vi "界面UI.vi"() -> ()   [LabVIEW 2016, in "超标留样集成.lvlib" / "ESTD1200.lvlib"]
uses:
  ESTD1200.lvlib
  <vilib>/Utility/miscctls.llb/LVPointTypeDef.ctl
  <vilib>/Plasmionique/MB Master/MB_Master/MB_Master.lvclass
  <vilib>/ptbypt/NI_PtbyPt.lvlib
  <vilib>/Plasmionique/MB Master/MB Master.lvlib
panel:
  in  "清除告警":bool
  in  "开门":bool
  out "采样瓶状态":T1
  out "冰箱温度":sgl
  out "瓶数":u16
  out "当前进程":u16(ring) items=["待机", "电机复位", "采样瓶转到采样区", "采样瓶排空", "采样泵管润洗", "采样瓶再排空", "采样", "采样泵反转排空管路", "取样瓶转到取样区"]
  out "流程计时/s":i32
  in  "设置":bool
  out "单次采样量":u16
  out "留样模式":enum16{"定时采样", "外控采样", "时间等比", "流量等比", "液位等比"}(ring)
  out "门状态":enum16{"门开", "门关"}(ring)
  out "报警状态":T2(ring)
  out "仪器时间":timestamp format="%<%Y/%m/%d %H:%M:%S>T"
  out "当前瓶号":u16
  out "采样器状态":enum16{"空闲", "忙碌"}(ring)
  out "采样器进程":i32(listbox)
  out "流程中":bool
  in  "停止流程":bool
  in  "启动流程":bool
  in  "远程复位":bool
  in  "远程留样":bool
  in  "停止命令":bool
  out "通讯":bool
  # "德润DR803L超标留样"
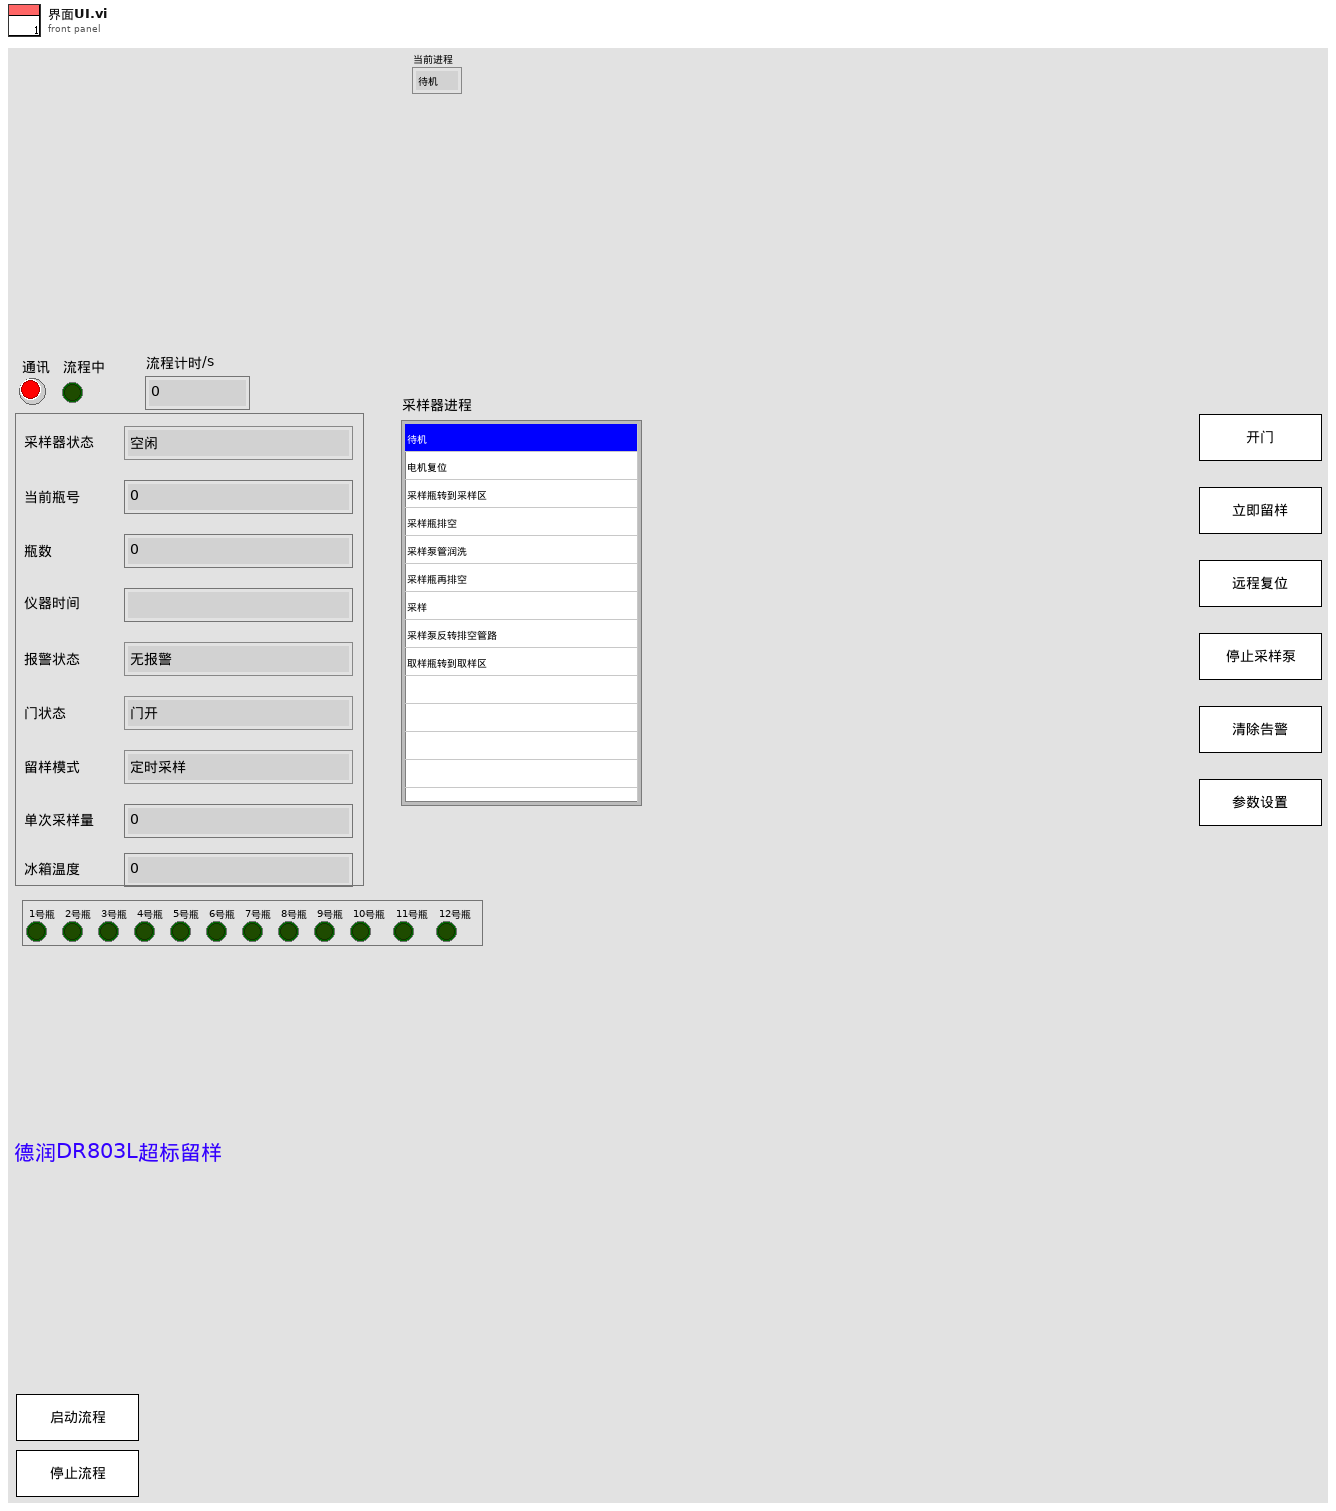
[diagram p1: front panel]
types:
  T1 = typedef "留样瓶状态.ctl" = cluster{"1号瓶":bool, "2号瓶":bool, "3号瓶":bool, "4号瓶":bool, "5号瓶":bool, "6号瓶":bool, "7号瓶":bool, "8号瓶":bool, "9号瓶":bool, "10号瓶":bool, "11号瓶":bool, "12号瓶":bool}
  T2 = enum16{"无报警", "通讯异常(采样器与工控机通讯)", "滑台电机异常(过温/过流)", "蠕动泵异常(过温/过流)", "转盘电机异常(过温/过流)", "编码器异常", "转盘原点传感器异常", "滑台原点传感器异常", "冰箱温度异常", "冰箱通讯异常", "门禁锁异常", "串口屏通信异常", "SD卡异常告警", "Flash异常告警(W25Q32)", "留样失败", "瓶满告警", "复位异常"}
  T3 = typedef "队列data.ctl" = cluster{"命令":string, "data":cluster{"站号":u16, "控制命令":u16[]}}
  T4 = cluster{"STEP":enum16{"open", "read", "write", "write single", "close"}, "starting address":u16, "value":u16}
  T5 = typedef "LVPointTypeDef.ctl" = cluster{"Horizontal":i16, "Vertical":i16}
  T6 = cluster{"命令":string, "data":cluster{"站号":u16, "控制命令":u16[]}}
  T7 = enum16{"open", "read", "write", "write single", "close"}
  T8 = enum32{"Bad", "Idle", "Run top level", "Running"}
  T9 = cluster{"当前瓶号":u16, "瓶数":u16, "采样量":u16, "采样模式":u16, "整点定时时间":cluster{"1":bool, "2":bool, "3":bool, "4":bool, "5":bool, "6":bool, "7":bool, "8":bool, "9":bool, "10":bool, "11":bool, "12":bool, "13":bool, "14":bool, "15":bool, "16":bool, "17":bool, "19":bool, "19":bool, "20":bool, "21":bool, "22":bool, "23":bool, "24":bool}, "氨氮":sgl, "总磷":sgl, "总氮":sgl, "CODMn":sgl, "CODCr":sgl, "PH":sgl, "溶解氧":sgl, "时间等比采样间隔":u16, "流量等比采样间隔":sgl, "4mA流量":sgl, "20mA流量":sgl, "当前流量":sgl, "液位等比采样间隔":sgl, "4mA液位":sgl, "20mA液位":sgl, "当前液位":sgl}
  T10 = cluster{"1":bool, "2":bool, "3":bool, "4":bool, "5":bool, "6":bool, "7":bool, "8":bool, "9":bool, "10":bool, "11":bool, "12":bool, "13":bool, "14":bool, "15":bool, "16":bool, "17":bool, "19":bool, "19":bool, "20":bool, "21":bool, "22":bool, "23":bool, "24":bool}
  T11 = cluster{"采样器状态":u16, "采样模式":u16, "瓶数":u16, "采样量":u16, "当前瓶号":u16, "当前进程":u16, "采样瓶状态":cluster{"1号瓶":bool, "2号瓶":bool, "3号瓶":bool, "4号瓶":bool, "5号瓶":bool, "6号瓶":bool, "7号瓶":bool, "8号瓶":bool, "9号瓶":bool, "10号瓶":bool, "11号瓶":bool, "12号瓶":bool}, "门锁状态":bool, "冰箱当前温度":sgl, "系统时间":timestamp}
  T12 = cluster{"系统时间":timestamp, "当前进程":u16, "采样模式":u16, "告警代码":u16, "故障代码":u16, "软件版本":string}
  T13 = cluster{"1号瓶":bool, "2号瓶":bool, "3号瓶":bool, "4号瓶":bool, "5号瓶":bool, "6号瓶":bool, "7号瓶":bool, "8号瓶":bool, "9号瓶":bool, "10号瓶":bool, "11号瓶":bool, "12号瓶":bool}
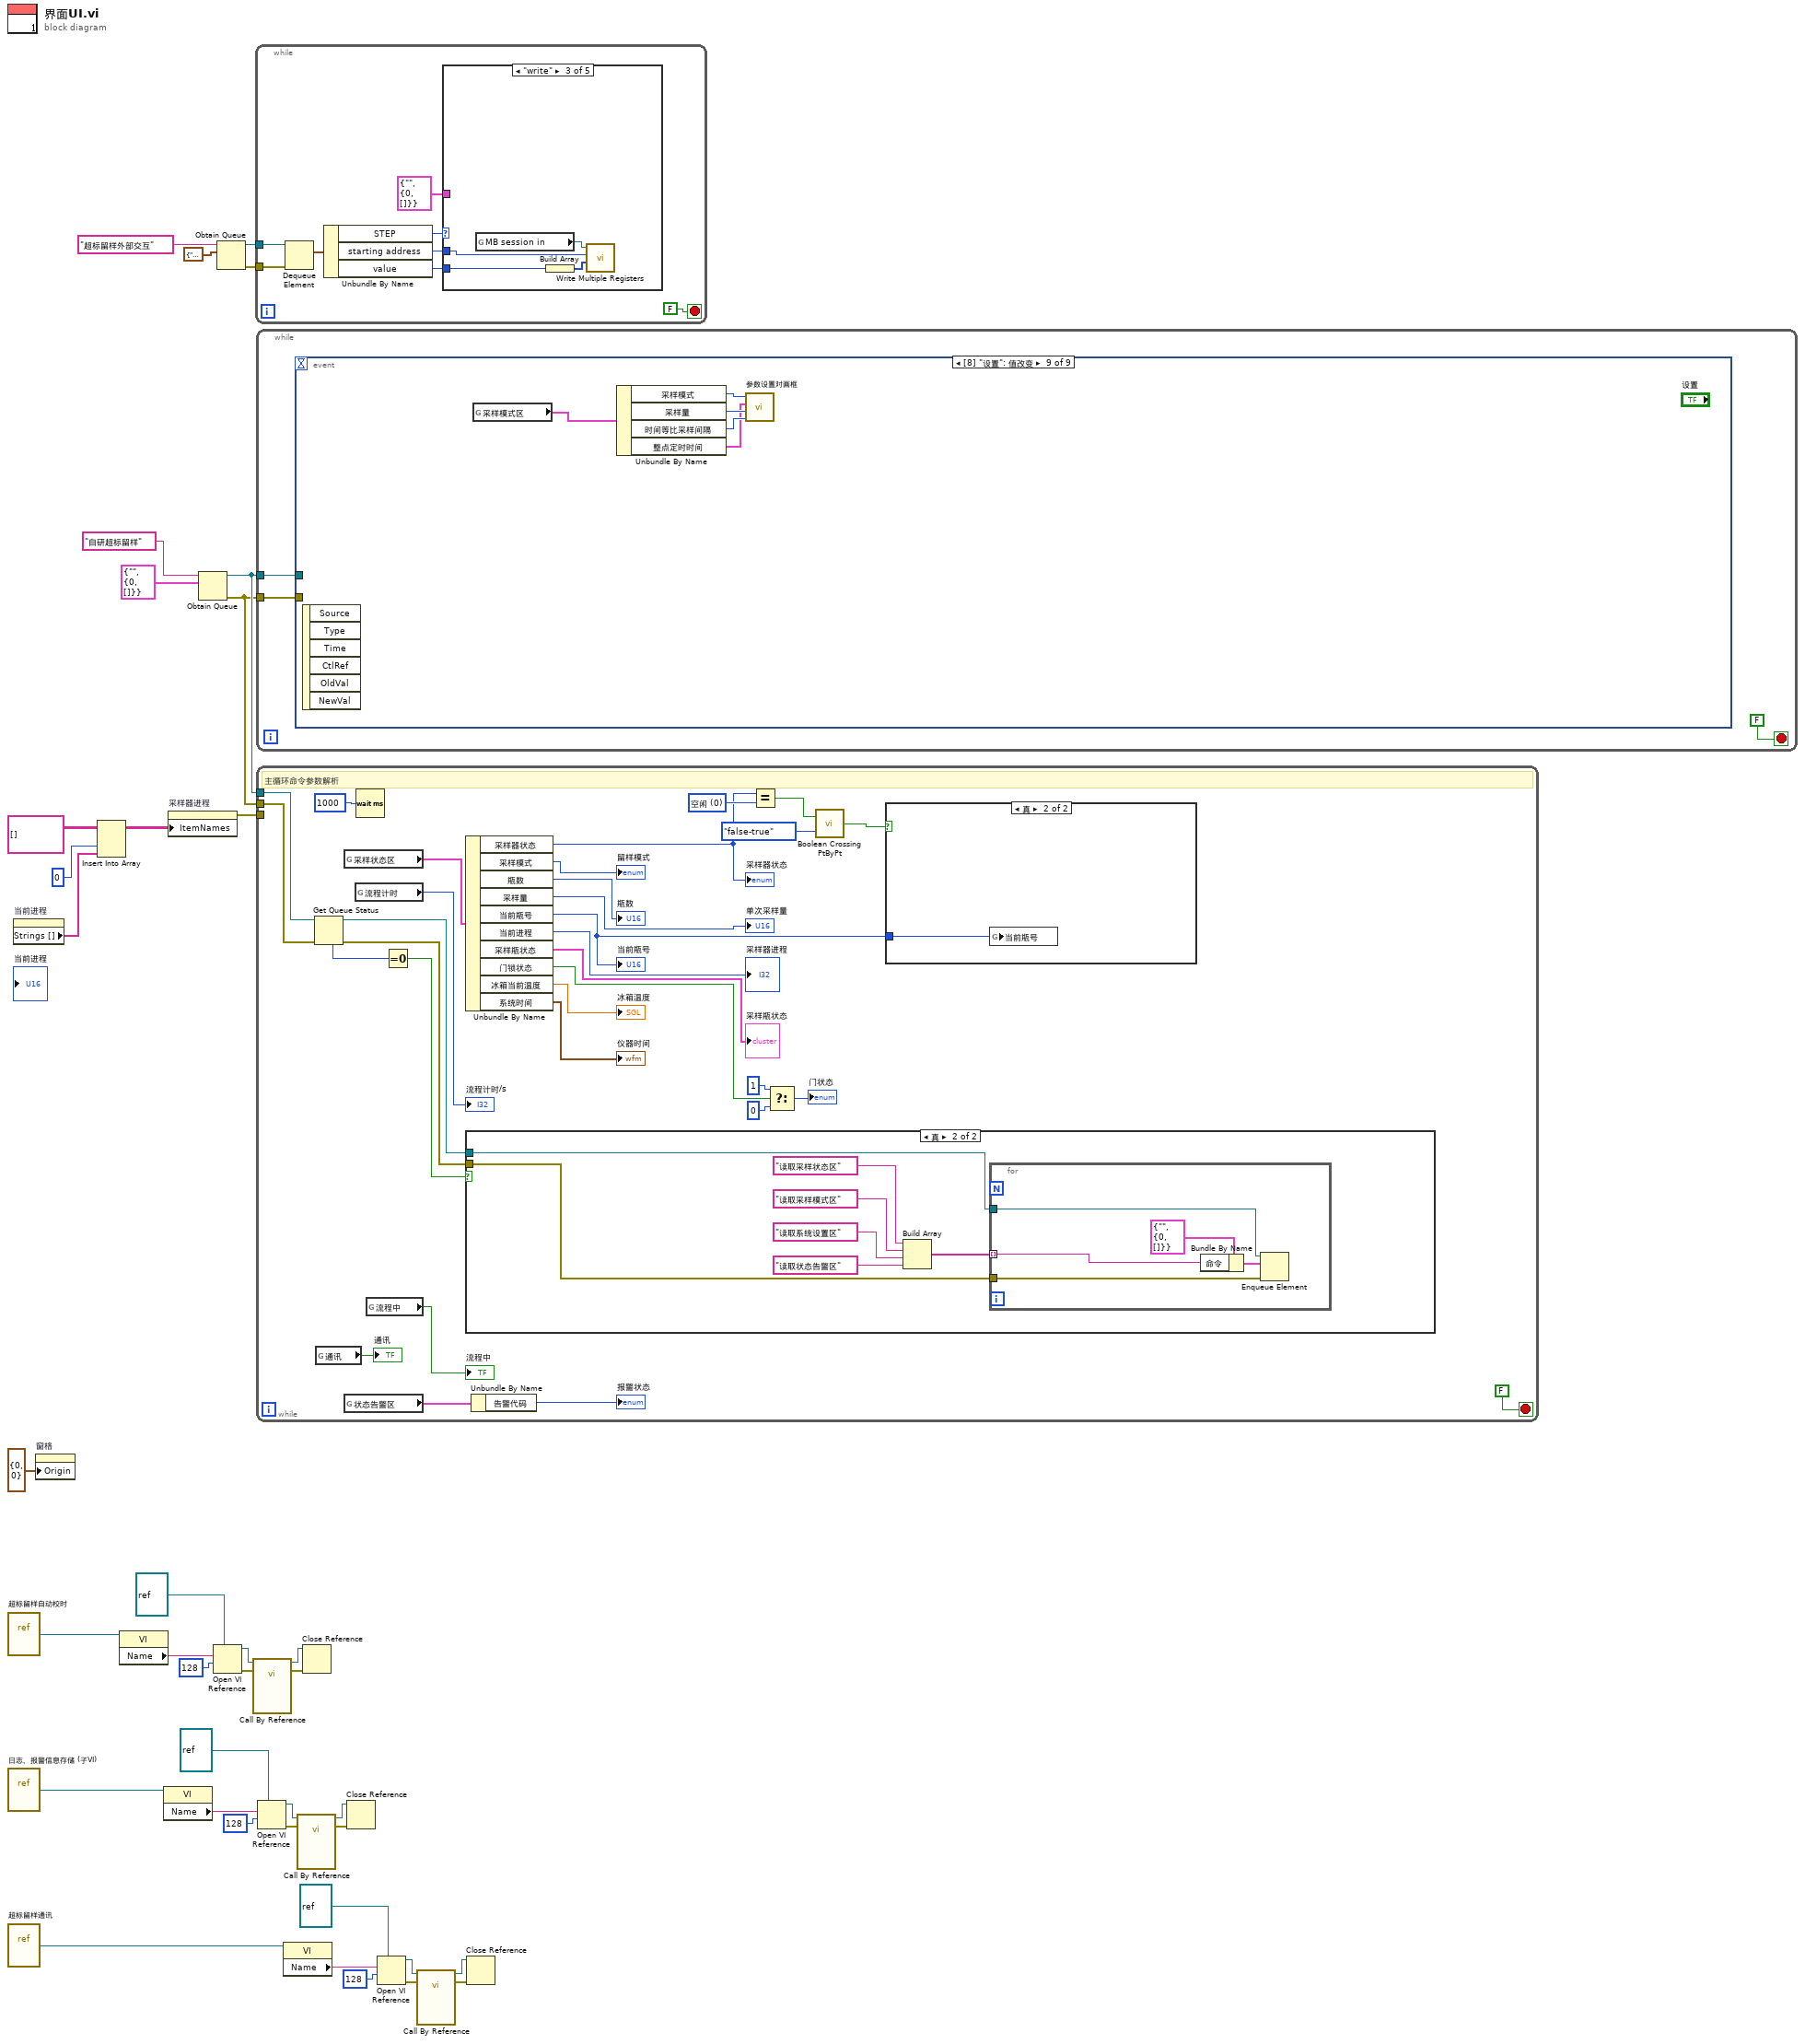
[diagram p0: block diagram]
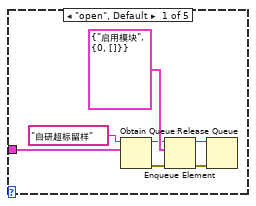
[diagram p2: hidden frame]
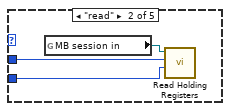
[diagram p3: hidden frame]
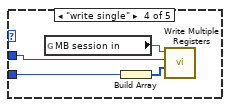
[diagram p4: hidden frame]
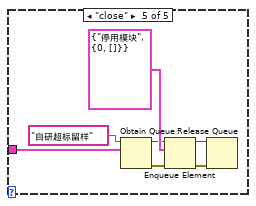
[diagram p5: hidden frame]
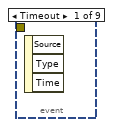
[diagram p6: hidden frame]
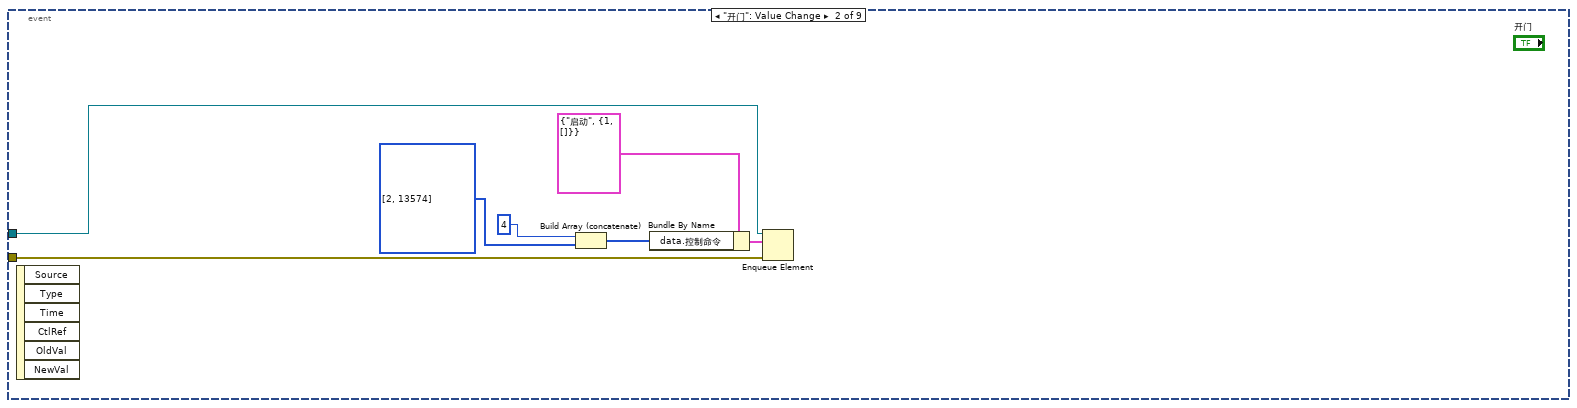
[diagram p7: hidden frame]
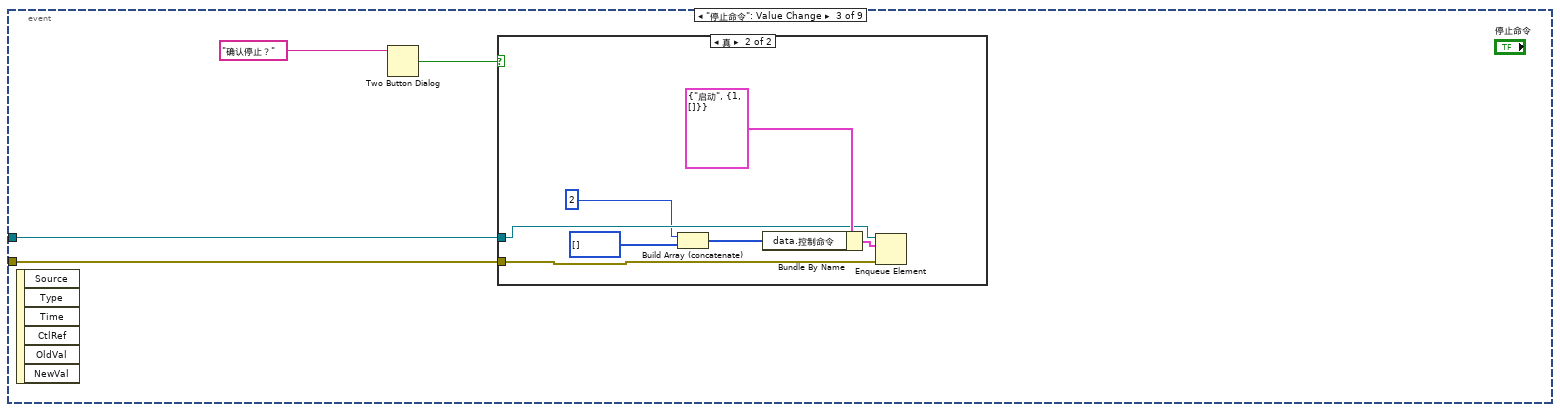
[diagram p8: hidden frame]
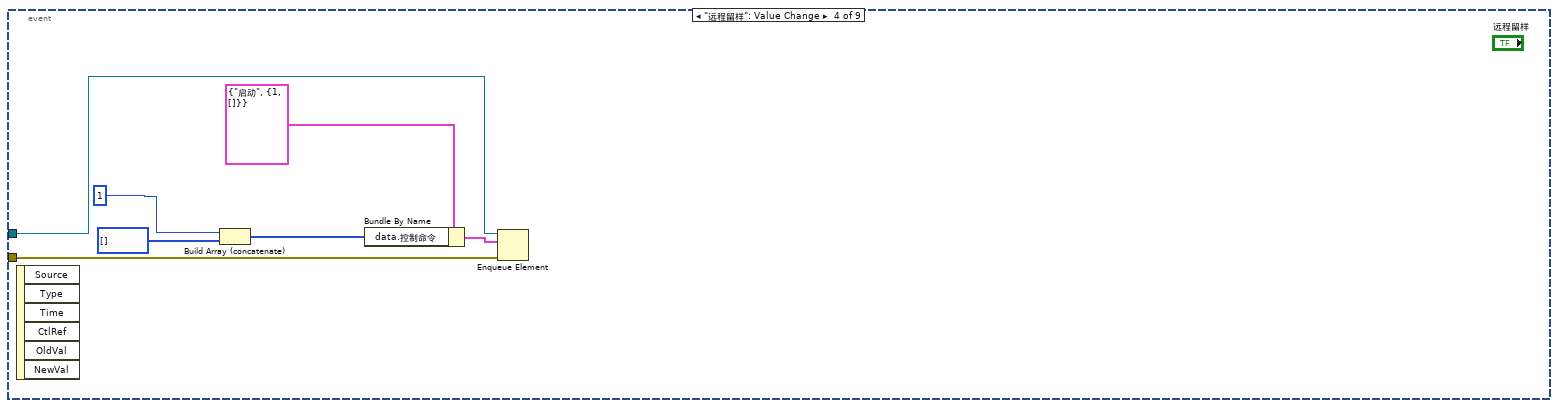
[diagram p10: hidden frame]
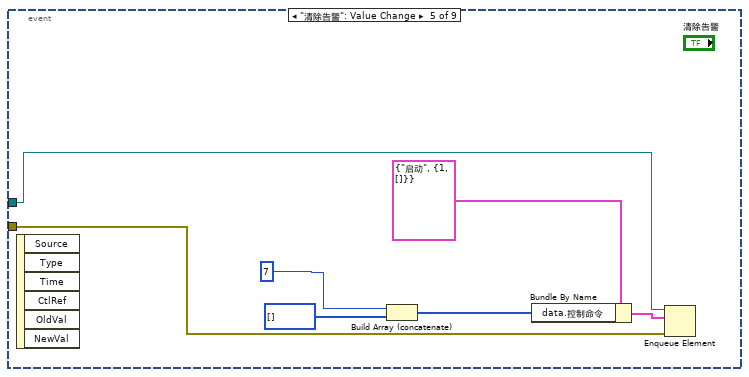
[diagram p11: hidden frame]
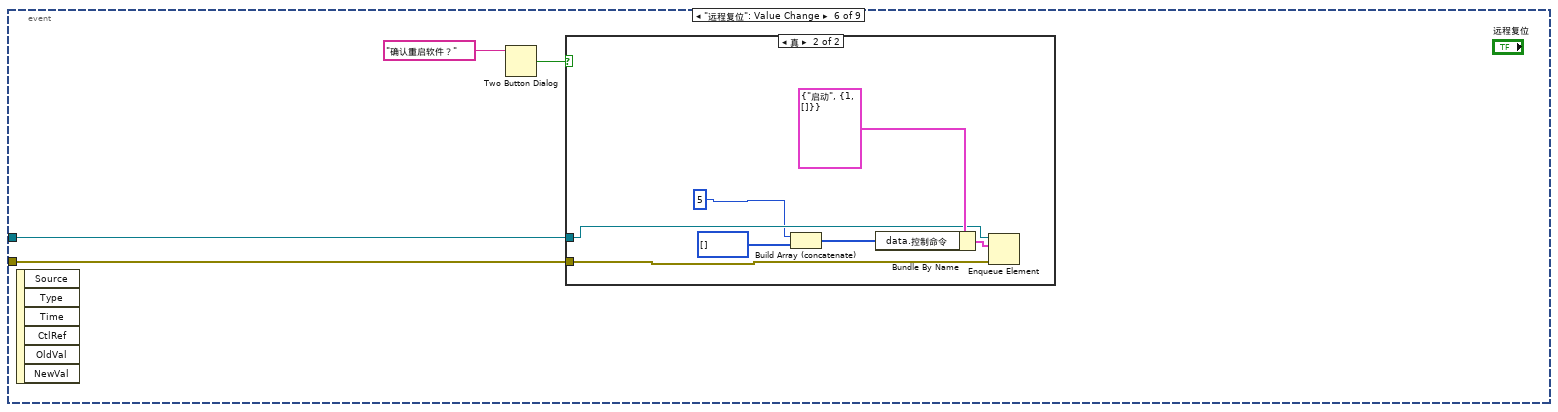
[diagram p12: hidden frame]
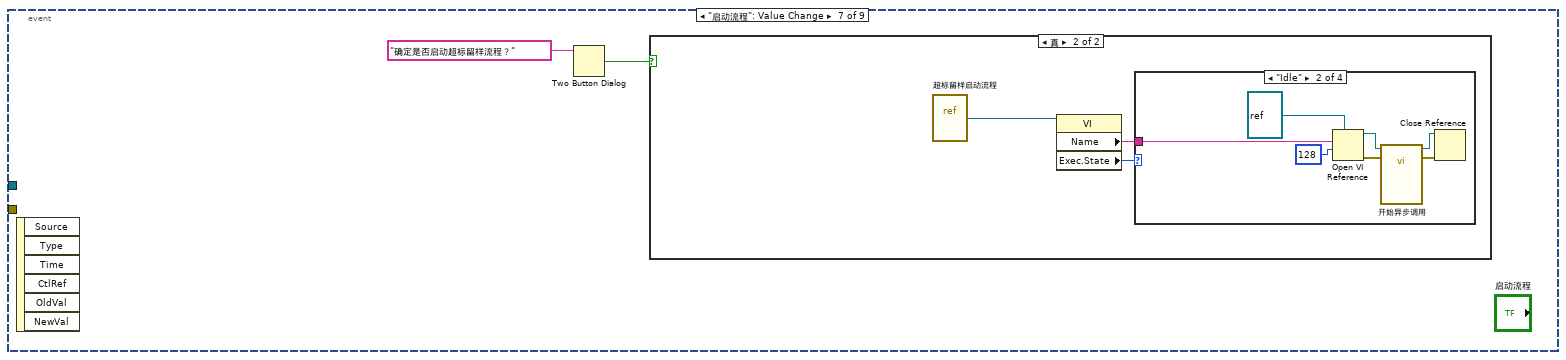
[diagram p14: hidden frame]
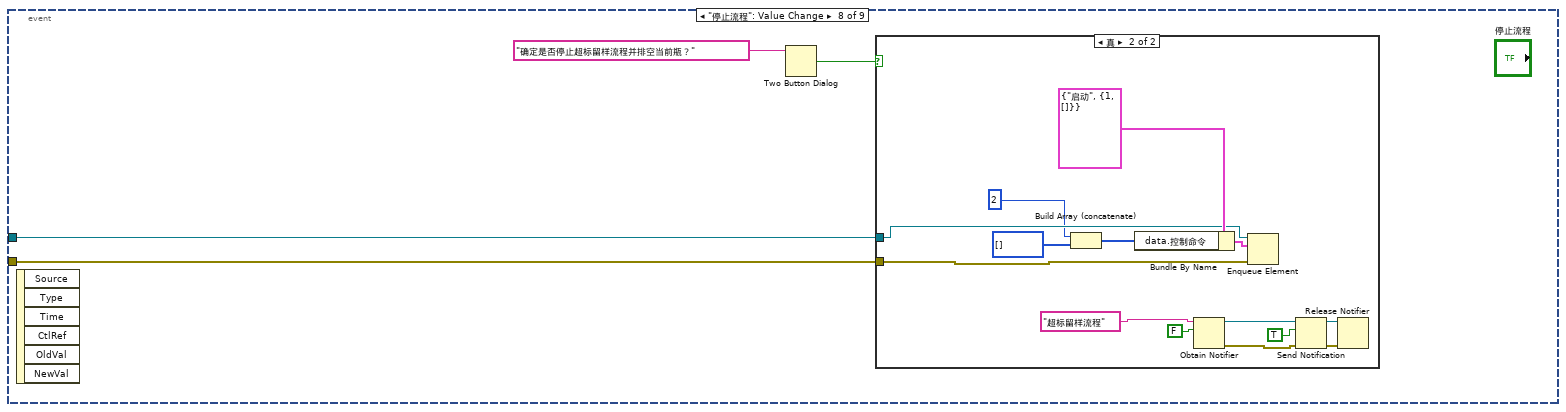
[diagram p19: hidden frame]
diagram:
  n1 = vi-ref "超标留样自动校时.vi"() -> (w25:refnum<vi>)
  n2 = vi-ref "日志、报警信息存储 (子VI).vi"() -> (w26:refnum<vi>)
  n3 = vi-ref "超标留样通讯.vi"() -> (w13:refnum<vi>)
  n4 = property on="当前进程" class="Ring (严格)"() -> ("Strings []"=w1:string[])  [unwired: 2 in, 2 out]
  n5 = property on="窗格" class="Pane"("Origin"=T5 {"Horizontal"=0, "Vertical"=0} ("原点")) -> ()  [unwired: 2 in, 2 out]
  n6 = Insert Into Array(array=string[][] [] ("字符串[]"), index (col)=0 ("禁用的索引 (列)"), new element=w1) -> (w15:string[][])  [unwired: 1 in]
  n7 = property class="VI"(reference=w25) -> ("Name"=w24:string)  [unwired: 1 in, 2 out]
  n8 = property class="VI"(reference=w26) -> ("Name"=w27:string)  [unwired: 1 in, 2 out]
  n9 = property on="采样器进程" class="MCListbox (严格)"("ItemNames"=w15) -> (error out=w14:errorcluster)  [unwired: 2 in, 1 out]
  n10 = Obtain Queue(name (unnamed)="自研超标留样" ("名称（未命名）"), element data type=T3 {"命令"="", "data"={"站号"=0, "控制命令"=[]}}) -> (queue out=w3:refnum<queue>, error out=w2:errorcluster)  [unwired: 3 in, 1 out]
  n11 = Open VI Reference(type specifier VI Refnum (for type only)=refnum<vi> refnum, vi path=w24, options=128 ("选项")) -> (vi reference=w22:refnum<vi>, error out=w20:errorcluster)  [unwired: 3 in]
  n12 = Obtain Queue(name (unnamed)="超标留样外部交互" ("名称（未命名）"), element data type=T4 {"STEP"=enum."write single", "starting address"=0, "value"=0}) -> (queue out=w35:refnum<queue>, error out=w34:errorcluster)  [unwired: 3 in, 1 out]
  n13 = call-by-ref "?"(reference=w22, error in=w20) -> (reference out=w18:refnum<vi>, error out=w19:errorcluster)  [unwired: 12 in]
  n14 = while {
    tunnel: w35 -> [w45]
    tunnel: w34 -> [w44]
    stop <- FALSE stop-if-true
    n15 = Dequeue Element(queue=w45, error in (no error)=w44) -> (element=w43:T4)  [unwired: 1 in, 3 out]
    n16 = Unbundle By Name(w43) -> ("STEP"=w42:T7, "starting address"=w41:u16, "value"=w40:u16)
    n17 = case shown="\"write\"" w42 {
      tunnel: w41 -> [_ w55 w59 w63 _]
      tunnel: w40 -> [_ w54 w57 w62 _]
      tunnel: T3 {"命令"="", "data"={"站号"=0, "控制命令"=[]}} -> [w47 _ _ _ w65]
      frame "open", Default {
        n18 = Obtain Queue(name (unnamed)="自研超标留样" ("名称（未命名）"), element data type=w47) -> (queue out=w51:refnum<queue>, error out=w50:errorcluster)  [unwired: 3 in, 1 out]
        n19 = Enqueue Element(queue=w51, element=T6 {"命令"="启用模块", "data"={"站号"=0, "控制命令"=[]}} ("元素"), error in (no error)=w50) -> (queue out=w49:refnum<queue>, error out=w48:errorcluster)  [unwired: 1 in, 1 out]
        n20 = Release Queue(queue=w49, error in (no error)=w48) -> ()  [unwired: 1 in, 3 out]
      }
      frame "read" {
        n21 = global read "超标留样全局.vi" "MB session in"() -> (w56:refnum<class "MB_Master.lvclass">)
        n22 = call <vilib>:"Read Holding Registers.vi"("quantity"=w54, "starting address"=w55, "MB session in"=w56) -> ()  [unwired: 6 in, 3 out]
      }
      frame "write" {
        n23 = global read "超标留样全局.vi" "MB session in"() -> (w60:refnum<class "MB_Master.lvclass">)
        n24 = Build Array(w57) -> (w58:u16[])
        n25 = call <vilib>:"Write Multiple Registers.vi"("values"=w58, "starting address"=w59, "MB session in"=w60) -> ()  [unwired: 7 in, 2 out]
      }
      frame "write single" {
        n26 = global read "超标留样全局.vi" "MB session in"() -> (w64:refnum<class "MB_Master.lvclass">)
        n27 = Build Array(w62) -> (w61:u16[])
        n28 = call <vilib>:"Write Multiple Registers.vi"("values"=w61, "starting address"=w63, "MB session in"=w64) -> ()  [unwired: 7 in, 2 out]
      }
      frame "close" {
        n29 = Obtain Queue(name (unnamed)="自研超标留样" ("名称（未命名）"), element data type=w65) -> (queue out=w69:refnum<queue>, error out=w68:errorcluster)  [unwired: 3 in, 1 out]
        n30 = Enqueue Element(queue=w69, element=T6 {"命令"="停用模块", "data"={"站号"=0, "控制命令"=[]}} ("元素"), error in (no error)=w68) -> (queue out=w67:refnum<queue>, error out=w66:errorcluster)  [unwired: 1 in, 1 out]
        n31 = Release Queue(queue=w67, error in (no error)=w66) -> ()  [unwired: 1 in, 3 out]
      }
    }
  }
  n32 = while {
    tunnel: w3 -> [w73]
    tunnel: w2 -> [w72]
    stop <- FALSE stop-if-true
    n33 = event shown="[8] \"设置\": 值改变" {
      selector: _ -> [_ _ _ _ _ _ _ _ _]
      dyn-events: _ -> [_ _ _ _ _ _ _ _ _]
      timeout: _ -> [_ _ _ _ _ _ _ _ _]
      tunnel: w73 -> [_ w77 w83 w95 w101 w108 _ w131 _]
      tunnel: w72 -> [_ w76 w82 w94 w100 w107 _ w130 _]
      event Timeout {
        n34 = event-data() -> ()  [unwired: 1 in, 3 out]
      }
      event "开门": Value Change {
        n35 = event-data() -> ()  [unwired: 1 in, 6 out]
        n36 = Build Array (concatenate)(u16 4 ("数值"), u16[] [2, 13574] ("控制命令")) -> (w79:u16[])
        n37 = Bundle By Name(cluster=T6 {"命令"="启动", "data"={"站号"=1, "控制命令"=[]}} ("元素"), "data.控制命令"=w79) -> (w78:T6)
        n38 = Enqueue Element(queue=w77, element=w78, error in (no error)=w76) -> ()  [unwired: 1 in, 3 out]
      }
      event "停止命令": Value Change {
        n39 = event-data() -> ()  [unwired: 1 in, 6 out]
        n40 = Two Button Dialog(message="确认停止？" ("消息")) -> (T button?=w84:bool)  [unwired: 2 in]
        n41 = case shown="真" w84 {
          tunnel: w83 -> [_ w88]
          tunnel: w82 -> [_ w87]
          frame False {
          }
          frame True {
            n42 = Build Array (concatenate)(u16 2 ("数值"), u16[] [] ("控制命令")) -> (w90:u16[])
            n43 = Bundle By Name(cluster=T6 {"命令"="启动", "data"={"站号"=1, "控制命令"=[]}} ("元素"), "data.控制命令"=w90) -> (w89:T6)
            n44 = Enqueue Element(queue=w88, element=w89, error in (no error)=w87) -> ()  [unwired: 1 in, 3 out]
          }
        }
      }
      event "远程留样": Value Change {
        n45 = event-data() -> ()  [unwired: 1 in, 6 out]
        n46 = Build Array (concatenate)(u16 1 ("数值"), u16[] [] ("控制命令")) -> (w97:u16[])
        n47 = Bundle By Name(cluster=T6 {"命令"="启动", "data"={"站号"=1, "控制命令"=[]}} ("元素"), "data.控制命令"=w97) -> (w96:T6)
        n48 = Enqueue Element(queue=w95, element=w96, error in (no error)=w94) -> ()  [unwired: 1 in, 3 out]
      }
      event "清除告警": Value Change {
        n49 = event-data() -> ()  [unwired: 1 in, 6 out]
        n50 = Build Array (concatenate)(u16 7 ("数值"), u16[] [] ("控制命令")) -> (w104:u16[])
        n51 = Bundle By Name(cluster=T6 {"命令"="启动", "data"={"站号"=1, "控制命令"=[]}} ("元素"), "data.控制命令"=w104) -> (w105:T6)
        n52 = Enqueue Element(queue=w101, element=w105, error in (no error)=w100) -> ()  [unwired: 1 in, 3 out]
      }
      event "远程复位": Value Change {
        n53 = event-data() -> ()  [unwired: 1 in, 6 out]
        n54 = Two Button Dialog(message="确认重启软件？" ("消息")) -> (T button?=w109:bool)  [unwired: 2 in]
        n55 = case shown="真" w109 {
          tunnel: w108 -> [_ w113]
          tunnel: w107 -> [_ w112]
          frame False {
          }
          frame True {
            n56 = Build Array (concatenate)(u16 5 ("数值"), u16[] [] ("控制命令")) -> (w115:u16[])
            n57 = Bundle By Name(cluster=T6 {"命令"="启动", "data"={"站号"=1, "控制命令"=[]}} ("元素"), "data.控制命令"=w115) -> (w114:T6)
            n58 = Enqueue Element(queue=w113, element=w114, error in (no error)=w112) -> ()  [unwired: 1 in, 3 out]
          }
        }
      }
      event "启动流程": Value Change {
        n59 = event-data() -> ()  [unwired: 1 in, 6 out]
        n60 = Two Button Dialog(message="确定是否启动超标留样流程？" ("消息")) -> (T button?=w118:bool)  [unwired: 2 in]
        n61 = case shown="真" w118 {
          frame False {
          }
          frame True {
            n62 = vi-ref "超标留样启动流程.vi"() -> (w120:refnum<vi>)
            n63 = property class="VI"(reference=w120) -> ("Name"=w121:string, "Exec.State"=w122:T8)  [unwired: 1 in, 2 out]
            n64 = case shown="\"Idle\"" w122 {
              tunnel: w121 -> [_ w125 _ _]
              frame "Bad", Default {
              }
              frame "Idle" {
                n65 = Open VI Reference(type specifier VI Refnum (for type only)=refnum<vi> refnum ("类型说明符VI引用句柄（仅用于类型）"), vi path=w125, options=128 ("选项")) -> (vi reference=w129:refnum<vi>, error out=w124:errorcluster)  [unwired: 3 in]
                n66 = call-by-ref "开始异步调用"(reference=w129, error in=w124) -> (reference out=w128:refnum<vi>, error out=w123:errorcluster)  [unwired: 12 in]
                n67 = Close Reference(reference=w128, error in (no error)=w123) -> ()  [unwired: 1 out]
              }
              frame "Run top level" {
              }
              frame "Running" {
              }
            }
          }
        }
      }
      event "停止流程": Value Change {
        n68 = event-data() -> ()  [unwired: 1 in, 6 out]
        n69 = Two Button Dialog(message="确定是否停止超标留样流程并排空当前瓶？" ("消息")) -> (T button?=w132:bool)  [unwired: 2 in]
        n70 = case shown="真" w132 {
          tunnel: w131 -> [_ w136]
          tunnel: w130 -> [_ w135]
          frame False {
          }
          frame True {
            n71 = Build Array (concatenate)(u16 2 ("数值"), u16[] [] ("控制命令")) -> (w138:u16[])
            n72 = Bundle By Name(cluster=T6 {"命令"="启动", "data"={"站号"=1, "控制命令"=[]}} ("元素"), "data.控制命令"=w138) -> (w137:T6)
            n73 = Obtain Notifier(name (unnamed)="超标留样流程" ("名称（未命名）"), notification data type=FALSE ("采样完成")) -> (notifier out=w145:refnum<notifier>, error out=w144:errorcluster)  [unwired: 2 in, 1 out]
            n74 = Enqueue Element(queue=w136, element=w137, error in (no error)=w135) -> ()  [unwired: 1 in, 3 out]
            n75 = Send Notification(notification=TRUE ("通知"), notifier=w145, error in (no error)=w144) -> (notifier out=w142:refnum<notifier>, error out=w141:errorcluster)
            n76 = Release Notifier(notifier=w142, error in (no error)=w141) -> ()  [unwired: 1 in, 3 out]
          }
        }
      }
      event "设置": Value Change {
        n77 = event-data() -> ()  [unwired: 1 in, 6 out]
        n78 = global read "超标留样全局.vi" "采样模式区"() -> (w152:T9)
        n79 = Unbundle By Name(w152) -> ("采样模式"=w151:u16, "采样量"=w150:u16, "时间等比采样间隔"=w149:u16, "整点定时时间"=w148:T10)
        n80 = call "参数设置对画框.vi"("时间等比采样"=w149, "单次采样量"=w150, "整点定时时间"=w148, "留样模式"=w151) -> ()  [unwired: 8 in]
      }
    }
  }
  n81 = while {
    tunnel: w3 -> [w181]
    tunnel: w2 -> [w180]
    tunnel: w14 -> [_]
    stop <- FALSE stop-if-true
    w166 = u16 0 items=["空闲", "忙碌"] ("采样器状态")
    # "主循环命令参数解析"
    n82 = Get Queue Status(queue=w181, error in (no error)=w180) -> (queue out=w178:refnum<queue>, error out=w177:errorcluster, # elements in queue=w179:i32)  [unwired: 1 in, 5 out]
    n83 = global read "超标留样全局.vi" "通讯"() -> (→"通讯":bool)
    n84 = global read "超标留样全局.vi" "采样状态区"() -> (w169:T11)
    n85 = global read "超标留样全局.vi" "状态告警区"() -> (w163:T12)
    n86 = global read "串口参数断电保存全局变量.vi" "流程计时"() -> (→"流程计时/s":i32)
    n87 = Wait (ms)(milliseconds to wait=u32 1000 ("等待时间（毫秒）")) -> ()  [unwired: 1 out]
    n88 = global read "串口参数断电保存全局变量.vi" "流程中"() -> (→"流程中":bool)
    n89 = Equal To 0?(x=w179) -> (x = 0?=w176:bool)
    n90 = Unbundle By Name(w169) -> ("采样器状态"=w165:u16, "采样模式"=→"留样模式":u16, "瓶数"=→"瓶数":u16, "采样量"=→"单次采样量":u16, "当前瓶号"=w167:u16, "当前进程"=→"采样器进程":u16, "采样瓶状态"=→"采样瓶状态":T13, "门锁状态"=w161:bool, "冰箱当前温度"=→"冰箱温度":sgl, "系统时间"=→"仪器时间":timestamp)
    "采样器状态" <- w165
    "当前瓶号" <- w167
    n91 = case shown="真" w176 {
      tunnel: w178 -> [_ w191]
      tunnel: w177 -> [_ w190]
      frame False {
      }
      frame True {
        n92 = Build Array("读取采样状态区" ("命令"), "读取采样模式区" ("命令"), "读取系统设置区" ("命令"), "读取状态告警区" ("命令")) -> (w188:string[])
        n93 = for {
          tunnel: w191 -> [w196]
          tunnel: w190 -> [w195]
          tunnel: w188 -> [w192] mode=indexing
          n94 = Bundle By Name(cluster=T3 {"命令"="", "data"={"站号"=0, "控制命令"=[]}}, "命令"=w192) -> (w193:T3)
          n95 = Enqueue Element(queue=w196, element=w193, error in (no error)=w195) -> ()  [unwired: 1 in, 3 out]
        }
      }
    }
    n96 = Unbundle By Name(w163) -> ("告警代码"=→"报警状态":u16)
    n97 = Equal?(x=w165, y=w166) -> (x = y?=w175:bool)
    n98 = Select(t=u16 1, s=w161, f=u16 0) -> (s? t:f=→"门状态":u16)
    n99 = call <vilib>:"Boolean Crossing PtByPt.vi"("direction"=enum16{"either", "false-true", "true-false"}."false-true", "input"=w175) -> ("crossing"=w173:bool)  [unwired: 1 in]
    n100 = case shown="真" w173 {
      tunnel: w167 -> [_ w184]
      frame False {
      }
      frame True {
        n101 = global write "超标留样全局.vi" "当前瓶号"(w184) -> ()
      }
    }
  }
  n102 = Open VI Reference(type specifier VI Refnum (for type only)=refnum<vi> refnum, vi path=w27, options=128 ("选项")) -> (vi reference=w29:refnum<vi>, error out=w31:errorcluster)  [unwired: 3 in]
  n103 = property class="VI"(reference=w13) -> ("Name"=w12:string)  [unwired: 1 in, 2 out]
  n104 = call-by-ref "?"(reference=w29, error in=w31) -> (reference out=w33:refnum<vi>, error out=w32:errorcluster)  [unwired: 12 in]
  n105 = Close Reference(reference=w18, error in (no error)=w19) -> ()  [unwired: 1 out]
  n106 = Close Reference(reference=w33, error in (no error)=w32) -> ()  [unwired: 1 out]
  n107 = Open VI Reference(type specifier VI Refnum (for type only)=refnum<vi> refnum, vi path=w12, options=128 ("选项")) -> (vi reference=w10:refnum<vi>, error out=w8:errorcluster)  [unwired: 3 in]
  n108 = call-by-ref "?"(reference=w10, error in=w8) -> (reference out=w6:refnum<vi>, error out=w7:errorcluster)  [unwired: 10 in, 2 out]
  n109 = Close Reference(reference=w6, error in (no error)=w7) -> ()  [unwired: 1 out]
